vi "Serial Write.vi"(8 "error in (no error)":errorcluster {"code" format="%.0x"}, 10 "Write Buffer (\"\")":string, 11 "VISA resource name":refnum<visa-resource-name>) -> (0 "error out":errorcluster {"code" format="%.0x"}, 2 "Return Count":u32, 3 "VISA resource name out":refnum<visa-resource-name>)   [LabVIEW 2019, in "Lake Shore Cryotronics 370.lvlib"]
doc: "This VI appends the carriage return, line feed characters \"\\r\\n\" to the end of the input string and writes the new string to the instrument."
uses:
  Lake Shore Cryotronics 370.lvlib
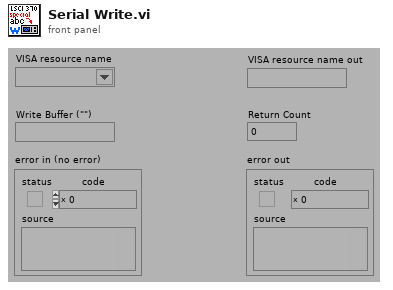
[diagram p1: front panel]
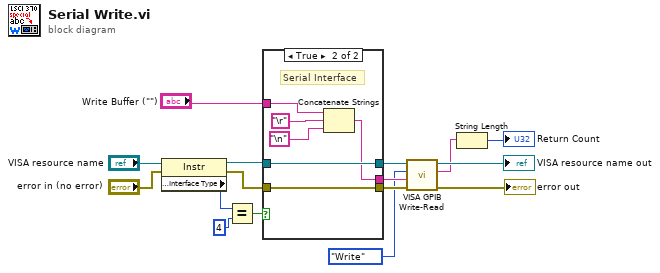
[diagram p0: block diagram]
diagram:
  n1 = property class="Instr"(reference="VISA resource name", error in="error in (no error)") -> (reference out=w12:refnum<visa-resource-name>, error out=w13:errorcluster, "Interface Information:Interface Type"=w10:u16)
  n2 = Equal?(x=w10, y=4) -> (x = y?=w9:bool)
  n3 = case shown="True" w9 {
    tunnel: [w17 w20] -> w5
    tunnel: [w18 w22] -> w4
    tunnel: w12 -> [w18 w22]
    tunnel: w13 -> [w17 w20]
    tunnel: "Write Buffer (\"\")" -> [w19 w25]
    tunnel: [w19 w21] -> w3
    frame False {
      # "GPIB Interface"
    }
    frame True {
      # "Serial Interface"
      n4 = Concatenate Strings(w25, "\r", "\n") -> (w21:string)
    }
  }
  n5 = call "VISA GPIB Write-Read.vi"("error in (no error)"=w5, "Command"=w3, "Action"=enum16{"Write", "Read", "Write & Read"}."Write", "VISA resource name"=w4) -> ("error out"=→"error out":errorcluster, "String Returned"=w7:string, "dup VISA Session"=→"VISA resource name out":refnum<visa-resource-name>)  [unwired: 4 in, 1 out]
  n6 = String Length(string=w7) -> (length=→"Return Count":i32)
